vi "UI.vi"(8 "error in (no error)":errorcluster) -> (0 "error out":errorcluster)   [LabVIEW 2018, in "Main.lvlib"]
uses:
  Main.lvlib
  Page/Page Action.ctl
  Page/Page.lvlib
  Page/Page Mouse.ctl
  <vilib>/Utility/miscctls.llb/LVPoint32TypeDef.ctl
  Page/Page Refnums.ctl
  Tab/Tab.lvlib
  Tab/Tab Action.ctl
  Tab/Tab Refnums.ctl
  Tab/Tab Mouse.ctl
  Page Log.vi
  Page Settings.vi
  Page Help.vi
  Page Packages.vi
  Page Network.vi
  Page Project.vi
  Page Getting Started.vi
panel:
  in  "Page Select":bool
  out "Page Picture":picture
  in  "Tab Select":bool
  out "Tab Picture":picture caption="Picture"
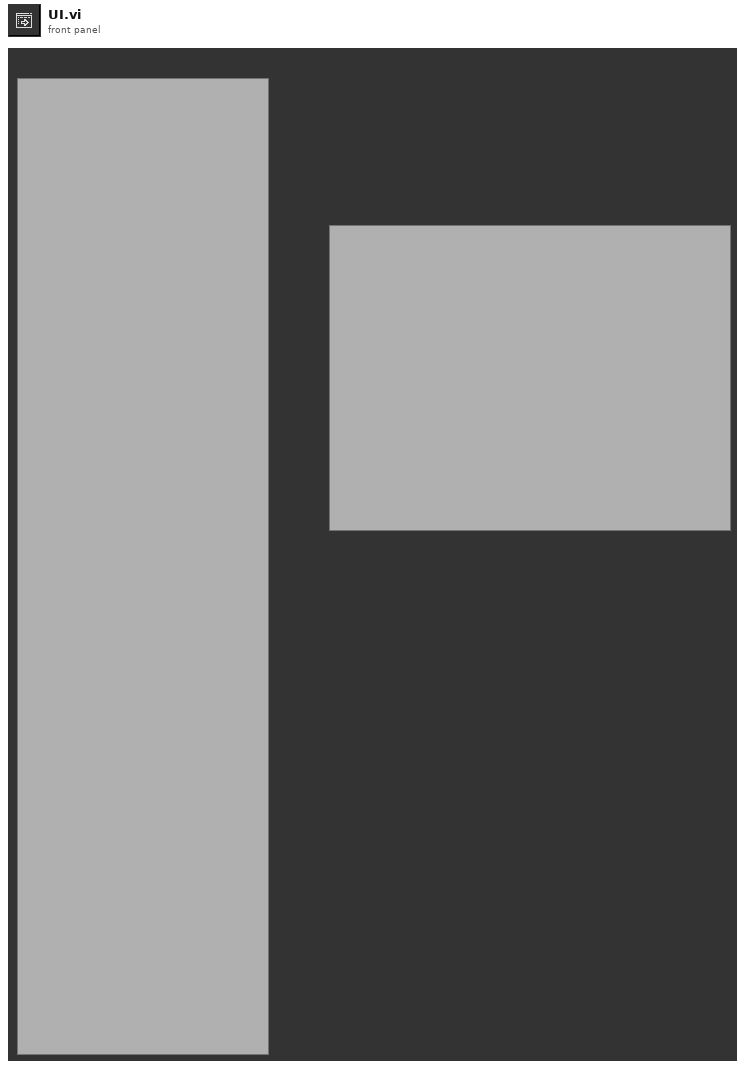
[diagram p1: front panel]
types:
  T1 = typedef "Page.lvlib/Page Action.ctl" = enum8{"noop", "new", "init", "close", "page_change", "page_hover", "render", "page_caption", "page_insert", "page_add", "start", "resize", "theme_change", "hide"}
  T2 = typedef "Tab.lvlib/Tab Action.ctl" = enum8{"noop", "new", "init", "close", "start", "render", "tab_add", "tab_change", "tab_hover", "tab_event", "tab_insert", "tab_popout", "tab_close", "theme_change", "resize"}
  T3 = typedef "Tab.lvlib/Tab Refnums.ctl" = cluster{"VI":refnum<vi>, "Picture":refnum<vi>, "Sub Panel":refnum<vi>}
  T4 = typedef "Page.lvlib/Page Refnums.ctl" = cluster{"VI Refnum":refnum<vi>, "Sub Panel":refnum<vi>, "Picture":refnum<vi>}
  T5 = typedef "Page.lvlib/Page Mouse.ctl" = cluster{"Horizontal":i32, "Vertical":i32, "Button":u16, "Shift":bool, "Ctrl":bool, "Alt":bool, "Double Click":bool}
  T6 = typedef "LVPoint32TypeDef.ctl" = cluster{"Horizontal":i32, "Vertical":i32}
  T7 = typedef "Tab.lvlib/Tab Mouse.ctl" = cluster{"Horizontal":i32, "Vertical":i32, "Button":u16, "Shift":bool, "Ctrl":bool, "Alt":bool, "Double Click":bool}
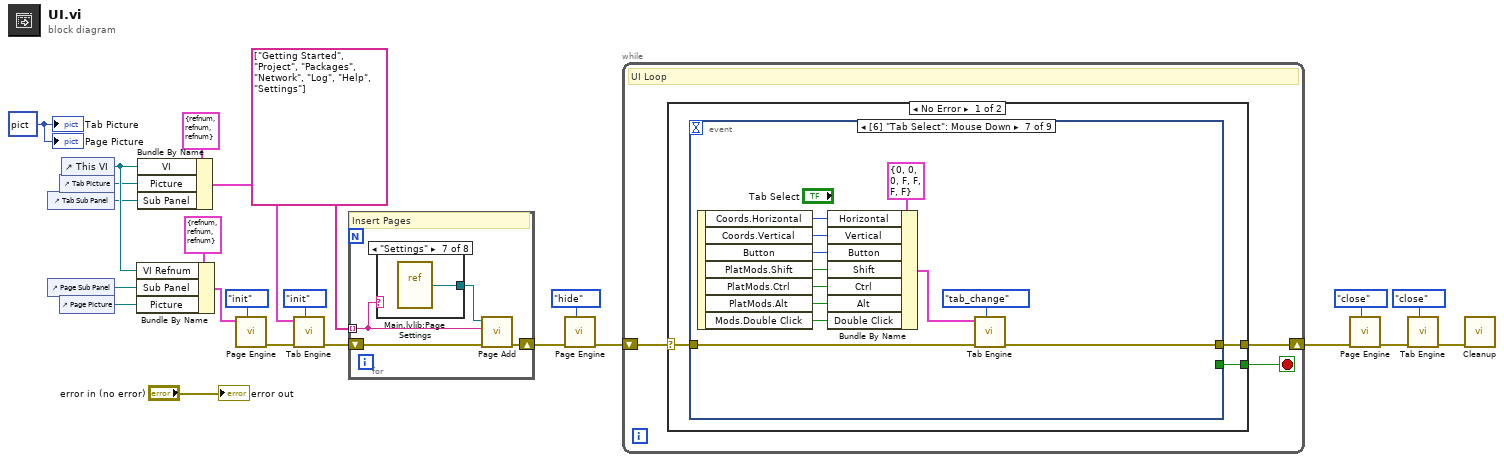
[diagram p0: block diagram]
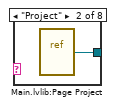
[diagram p3: hidden frame]
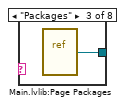
[diagram p4: hidden frame]
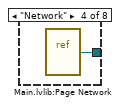
[diagram p5: hidden frame]
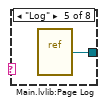
[diagram p6: hidden frame]
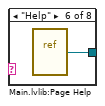
[diagram p7: hidden frame]
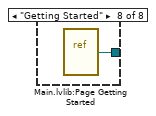
[diagram p8: hidden frame]
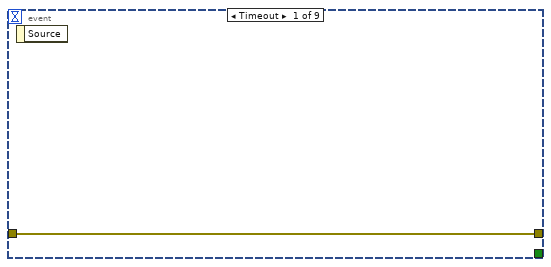
[diagram p9: hidden frame]
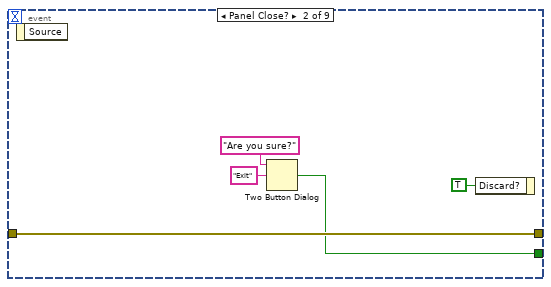
[diagram p10: hidden frame]
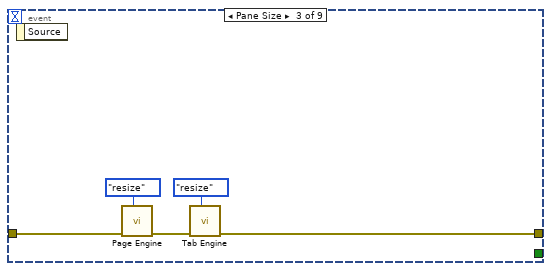
[diagram p11: hidden frame]
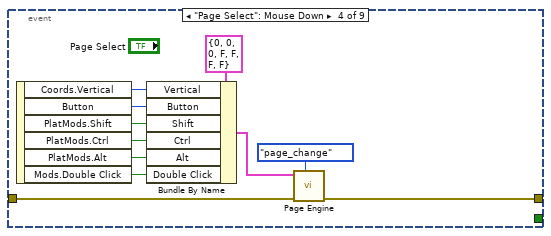
[diagram p12: hidden frame]
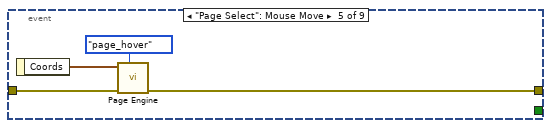
[diagram p13: hidden frame]
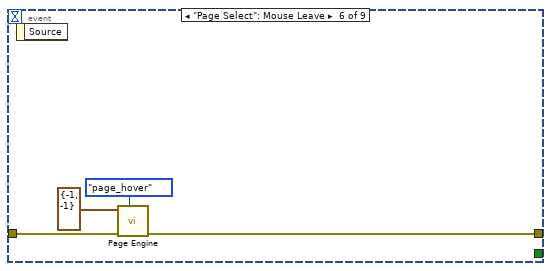
[diagram p14: hidden frame]
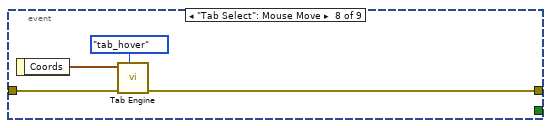
[diagram p15: hidden frame]
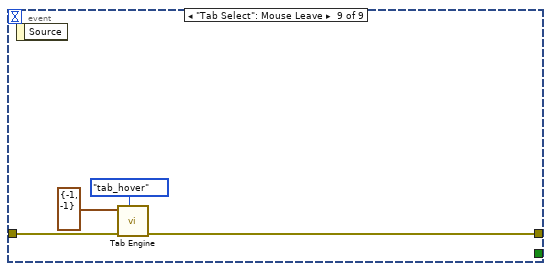
[diagram p16: hidden frame]
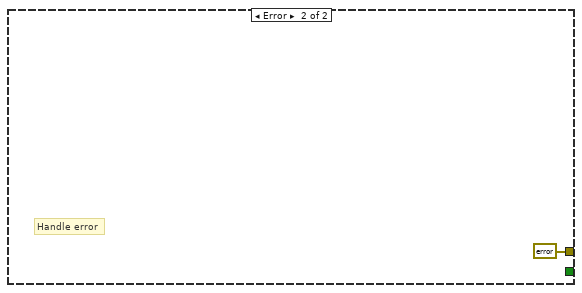
[diagram p17: hidden frame]
diagram:
  w7 = picture data[5B] ("Tab Picture")
  n1 = control-ref of="Tab Sub Panel"() -> (w12:refnum<vi>)
  n2 = control-ref of="Page Sub Panel"() -> (w20:refnum<vi>)
  n3 = control-ref of="Tab Picture"() -> (w13:refnum<vi>)
  n4 = control-ref of="Page Picture"() -> (w19:refnum<vi>)
  n5 = control-ref of="This VI"() -> (w14:refnum<vi>)
  n6 = Bundle By Name(cluster=T4 {"VI Refnum"=refnum, "Sub Panel"=refnum, "Picture"=refnum} ("Refnums"), "VI Refnum"=w14, "Sub Panel"=w20, "Picture"=w19) -> (w21:T4)
  n7 = Bundle By Name(cluster=T3 {"VI"=refnum, "Picture"=refnum, "Sub Panel"=refnum} ("Refnums"), "VI"=w14, "Picture"=w13, "Sub Panel"=w12) -> (w16:T3)
  n8 = call "Page Engine.vi"("Action"=Page_Action."init", "Data in"=w21) -> ("error out"=w15:errorcluster)  [unwired: 8 in, 1 out]
  n9 = call "Tab Engine.vi"("Action"=Tab_Action."init", "error in (no error)"=w15, "Variant in"=w16) -> ("error out"=w4:errorcluster)  [unwired: 7 in, 1 out]
  n10 = for {
    tunnel: string[] ["Getting Started", "Project", "Packages", "Network", "Log", "Help", "Settings"] -> [w27] mode=indexing
    shift-right: [w28] -> w2
    shift-left: w4 -> [w25]
    # "Insert Pages"
    n11 = case shown="\"Settings\"" w27 {
      tunnel: [_ w29 w30 w31 w32 w33 w34 w35] -> w26
      frame Default {
      }
      frame "Project" {
        n12 = vi-ref "Main.lvlib:Page Project.vi"() -> (w29:refnum<vi>)
      }
      frame "Packages" {
        n13 = vi-ref "Main.lvlib:Page Packages.vi"() -> (w30:refnum<vi>)
      }
      frame "Network" {
        n14 = vi-ref "Main.lvlib:Page Network.vi"() -> (w31:refnum<vi>)
      }
      frame "Log" {
        n15 = vi-ref "Main.lvlib:Page Log.vi"() -> (w32:refnum<vi>)
      }
      frame "Help" {
        n16 = vi-ref "Main.lvlib:Page Help.vi"() -> (w33:refnum<vi>)
      }
      frame "Settings" {
        n17 = vi-ref "Main.lvlib:Page Settings.vi"() -> (w34:refnum<vi>)
      }
      frame "Getting Started" {
        n18 = vi-ref "Main.lvlib:Page Getting Started.vi"() -> (w35:refnum<vi>)
      }
    }
    n19 = call "Page Add.vi"("error in (no error)"=w25, "Caption"=w27, "VI Refnum"=w26) -> ("error out"=w28:errorcluster)  [unwired: 8 in]
  }
  n20 = call "Page Engine.vi"("Action"=Page_Action."hide", "error in (no error)"=w2) -> ("error out"=w1:errorcluster)  [unwired: 8 in, 1 out]
  n21 = while {
    shift-right: [w36] -> w8
    shift-left: w1 -> [w37]
    stop <- w38 stop-if-true
    # "UI Loop"
    n22 = case shown="No Error" w37 {
      selector: w37 -> [w40 _]
      tunnel: [w41 _] -> w38
      tunnel: [w39 errorcluster {"status"=FALSE, "code"=0, "source"=""} ("error out")] -> w36
      frame No Error {
        n23 = event shown="[6] \"Tab Select\": Mouse Down" {
          selector: _ -> [_ _ _ _ _ _ _ _ _]
          dyn-events: _ -> [_ _ _ _ _ _ _ _ _]
          timeout: _ -> [_ _ _ _ _ _ _ _ _]
          tunnel: [_ w43 _ _ _ _ _ _ _] -> w41
          tunnel: w40 -> [w42 w46 w51 w62 w66 w70 w83 w87 w90]
          tunnel: [w42 w46 w48 w61 w65 w69 w82 w86 w89] -> w39
          event Timeout {
            n24 = event-data() -> ()  [unwired: 1 in, 1 out]
          }
          event Panel Close? {
            n25 = event-data() -> ()  [unwired: 1 in, 1 out]
            n26 = Two Button Dialog(message="Are you sure?", 2:"Exit" ("T button name (\"OK\")")) -> (T button?=w43:bool)  [unwired: 1 in]
            n27 = event-data("Discard?"=TRUE) -> ()  [unwired: 1 in, 1 out]
          }
          event Pane Size {
            n28 = event-data() -> ()  [unwired: 1 in, 1 out]
            n29 = call "Page Engine.vi"("Action"=Page_Action."resize", "error in (no error)"=w51) -> ("error out"=w49:errorcluster)  [unwired: 8 in, 1 out]
            n30 = call "Tab Engine.vi"("Action"=Tab_Action."resize", "error in (no error)"=w49) -> ("error out"=w48:errorcluster)  [unwired: 8 in, 1 out]
          }
          event "Page Select": Mouse Down {
            n31 = event-data() -> ("Coords.Vertical"=w58:i32, "Button"=w57:u16, "PlatMods.Shift"=w56:bool, "PlatMods.Ctrl"=w55:bool, "PlatMods.Alt"=w54:bool, "Mods.Double Click"=w53:bool)  [unwired: 1 in]
            n32 = Bundle By Name(cluster=T5 {"Horizontal"=0, "Vertical"=0, "Button"=0, "Shift"=FALSE, "Ctrl"=FALSE, "Alt"=FALSE, "Double Click"=FALSE} ("Page Mouse"), "Vertical"=w58, "Button"=w57, "Shift"=w56, "Ctrl"=w55, "Alt"=w54, "Double Click"=w53) -> (w59:T5)
            n33 = call "Page Engine.vi"("Action"=Page_Action."page_change", "error in (no error)"=w62, "Data in"=w59) -> ("error out"=w61:errorcluster)  [unwired: 7 in, 1 out]
          }
          event "Page Select": Mouse Move {
            n34 = event-data() -> ("Coords"=w64:T6)  [unwired: 1 in]
            n35 = call "Page Engine.vi"("Action"=Page_Action."page_hover", "error in (no error)"=w66, "Data in"=w64) -> ("error out"=w65:errorcluster)  [unwired: 7 in, 1 out]
          }
          event "Page Select": Mouse Leave {
            n36 = event-data() -> ()  [unwired: 1 in, 1 out]
            n37 = call "Page Engine.vi"("Action"=Page_Action."page_hover", "error in (no error)"=w70, "Data in"=T6 {"Horizontal"=-1, "Vertical"=-1} ("Coords")) -> ("error out"=w69:errorcluster)  [unwired: 7 in, 1 out]
          }
          event "Tab Select": Mouse Down {
            n38 = event-data() -> ("Coords.Horizontal"=w72:i32, "Coords.Vertical"=w79:i32, "Button"=w78:u16, "PlatMods.Shift"=w77:bool, "PlatMods.Ctrl"=w76:bool, "PlatMods.Alt"=w75:bool, "Mods.Double Click"=w74:bool)  [unwired: 1 in]
            n39 = Bundle By Name(cluster=T7 {"Horizontal"=0, "Vertical"=0, "Button"=0, "Shift"=FALSE, "Ctrl"=FALSE, "Alt"=FALSE, "Double Click"=FALSE} ("Page Mouse"), "Horizontal"=w72, "Vertical"=w79, "Button"=w78, "Shift"=w77, "Ctrl"=w76, "Alt"=w75, "Double Click"=w74) -> (w80:T7)
            n40 = call "Tab Engine.vi"("Action"=Tab_Action."tab_change", "error in (no error)"=w83, "Variant in"=w80) -> ("error out"=w82:errorcluster)  [unwired: 7 in, 1 out]
          }
          event "Tab Select": Mouse Move {
            n41 = event-data() -> ("Coords"=w85:T6)  [unwired: 1 in]
            n42 = call "Tab Engine.vi"("Action"=Tab_Action."tab_hover", "error in (no error)"=w87, "Variant in"=w85) -> ("error out"=w86:errorcluster)  [unwired: 7 in, 1 out]
          }
          event "Tab Select": Mouse Leave {
            n43 = event-data() -> ()  [unwired: 1 in, 1 out]
            n44 = call "Tab Engine.vi"("Action"=Tab_Action."tab_hover", "error in (no error)"=w90, "Variant in"=T6 {"Horizontal"=-1, "Vertical"=-1} ("Coords")) -> ("error out"=w89:errorcluster)  [unwired: 7 in, 1 out]
          }
        }
      }
      frame Error {
        # "Handle error"
      }
    }
  }
  n45 = call "Page Engine.vi"("Action"=Page_Action."close", "error in (no error)"=w8) -> ("error out"=w11:errorcluster)  [unwired: 8 in, 1 out]
  n46 = call "Tab Engine.vi"("Action"=Tab_Action."close", "error in (no error)"=w11) -> ("error out"=w6:errorcluster)  [unwired: 8 in, 1 out]
  n47 = call "Cleanup.vi"("error in (no error)"=w6) -> ()  [unwired: 10 in, 1 out]
  "error out" <- "error in (no error)"
  "Tab Picture" <- w7
  "Page Picture" <- w7
